vi "test_turbo1.vi"() -> ()   [LabVIEW 2018]
uses:
  <vilib>/addons/Modulation/Analog/support/mod_Set Error Source.vi
  <vilib>/addons/Modulation/Digital/Support/Common/Validators/mod_AWGN Validate.vi
  <vilib>/addons/Modulation/Digital/Impairments/subVIs/mod_createSeeds.vi
  <vilib>/addons/Modulation/Digital/Support/Common/Validators/mod_Validate Samples Per Symbol.vi
  <vilib>/addons/Modulation/Analog/support/Validators/mod_Validate Complex Waveform.vi
  <vilib>/addons/Modulation/Analog/support/Validators/mod_WFErrorHandler.vi
  <vilib>/addons/Modulation/Digital/Support/Common/Validators/mod_Generate Filter Coefficients Validate.vi
  <vilib>/addons/Modulation/Digital/General/subVIs/mod_Generate Filter Coefficients.vi
  <vilib>/addons/Modulation/Digital/General/MT Generate PSK System Parameters(M).vi
  <vilib>/addons/Modulation/Digital/General/subVIs/mod_Generate Bits PN Sequence.vi
  <vilib>/Analysis/1siggen.llb/Gaussian White Noise (obs 90).vi
  <vilib>/addons/Modulation/Digital/General/MT Apply Matched Filter (Generic).vi
  <vilib>/addons/Modulation/niDMT.lvlib
panel:
  out "size(s) 2":i32
  out "size(s)":i32
  out "%%%":i32
  out "****":i32
  out "ЁЁ":i32
  out "sortie turbocodeur":string
  out "BER":dbl
  in  "Eb/N0":dbl=10.0 format="%.2f"
  out "message":i8[](array[numeric])
  out "dec":i8[](array[numeric])
  out "sigma2":string
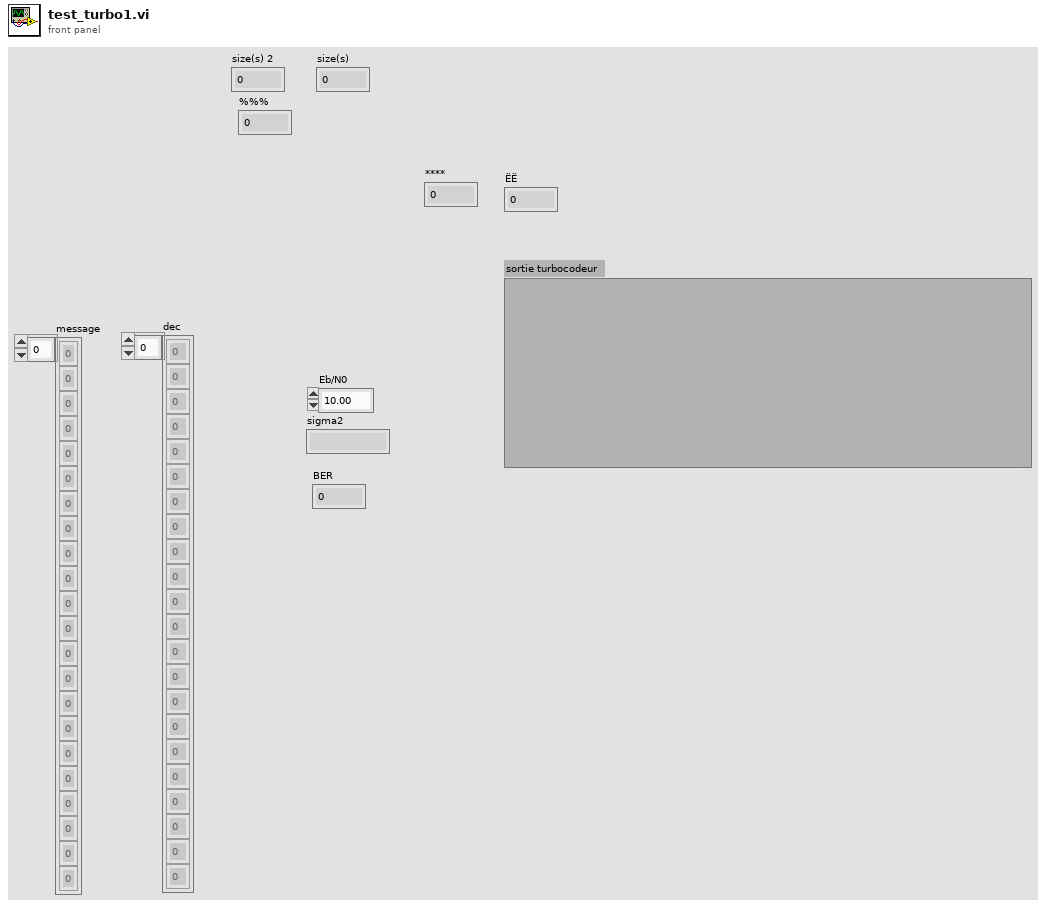
[diagram p1: front panel]
types:
  T1 = enum16{"none", "Raised Cosine", "Root Raised Cos", "Gaussian"}
  T2 = cluster{"samples per symbol (16)":i32, "symbol map":cdb[], "differential PSK":enum16{"disable", "enable"}, "PSK type":u16}
  T3 = typedef "niAMT.lvlib/Complex Data Waveform.ctl" = cluster{"t0":dbl, "dt":dbl, "Y":cdb[]}
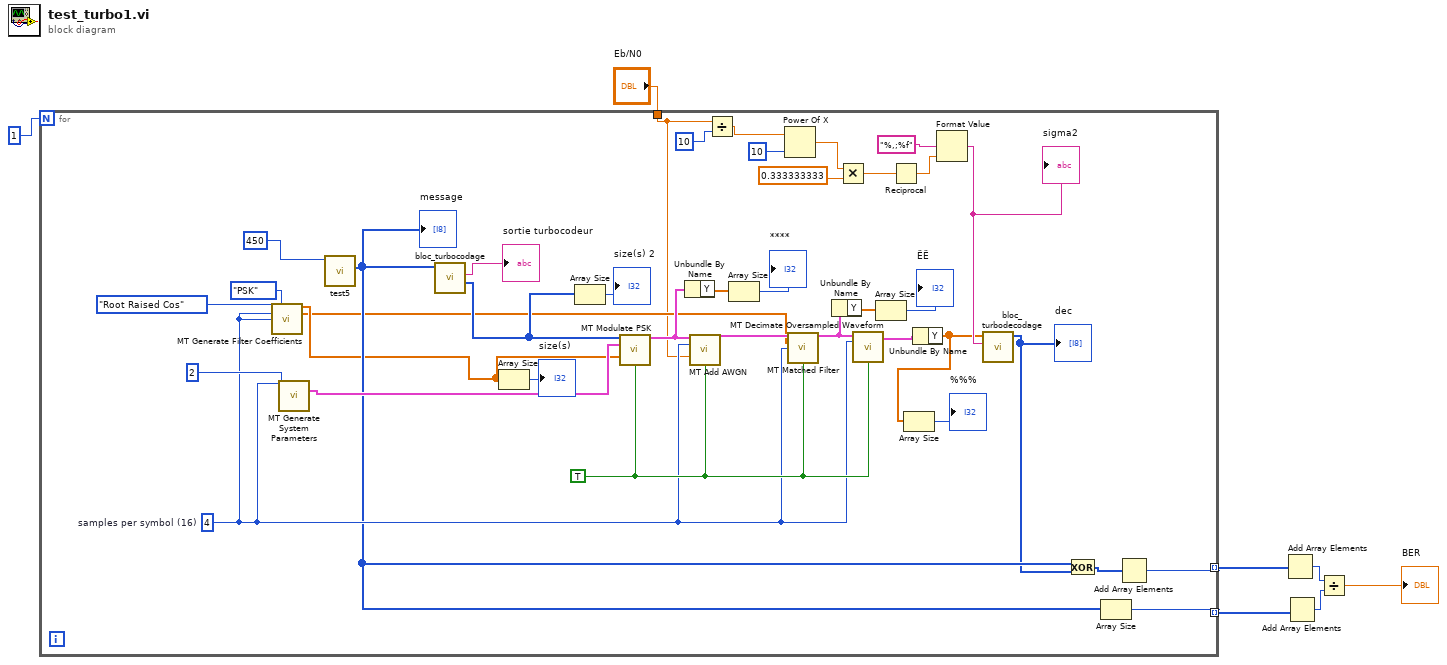
[diagram p0: block diagram]
diagram:
  n1 = for {
    N: 1 -> [_]
    tunnel: [w31] -> w5 mode=indexing
    tunnel: [w30] -> w4 mode=indexing
    tunnel: "Eb/N0" -> [w10]
    w38 = 4  # samples per symbol (16)
    w42 = TRUE ("reset? (T)")
    n2 = call <vilib>:"MT Generate Filter Coefficients.vi"("pulse shaping filter (none)"=T1."Root Raised Cos", "modulation type"=enum16{"FSK", "PSK", "QAM", "MSK", "PAM", "ASK"}."PSK", "pulse shaping samples per symbol (16)"=w38, "matched samples per symbol (16)"=w38) -> ("pulse shaping filter coefficients"=w16:dbl[], "matched filter coefficients"=w13:dbl[])  [unwired: 9 in, 1 out]
    n3 = call-poly <vilib>:"MT Generate System Parameters.vi"("samples per symbol (16)"=w38, "M-PSK (4)"=2) -> ("PSK system parameters"=w37:T2)  [unwired: 11 in, 2 out]
    n4 = call "test5.vi"("k"=450) -> ("output bit stream"=w29:i8[])  [unwired: 9 in, 1 out]
    "message" <- w29
    n5 = call "bloc_turbocodage.vi"("Array in"=w29) -> ("output bit stream"=w18:i8[], "sortie turbocodeur"=→"sortie turbocodeur":string)  [unwired: 8 in, 1 out]
    n6 = Array Size(array=w16) -> (size(s)=→"size(s)":i32)
    n7 = Array Size(array=w18) -> (size(s)=→"size(s) 2":i32)
    n8 = call <vilib>:"MT Modulate PSK.vi"("input bit stream"=w18, "PSK system parameters"=w37, "pulse shaping filter coefficients"=w16, "reset? (T)"=w42) -> ("output complex waveform"=w15:T3)  [unwired: 9 in, 2 out]
    n9 = Unbundle By Name(w15) -> ("Y"=w14:cdb[])
    n10 = call <vilib>:"MT Add AWGN.vi"("input complex waveform"=w15, "samples per symbol (16)"=w38, "Eb/N0 (10 dB)"=w10, "reset? (T)"=w42) -> ("output complex waveform"=w45:T3)  [unwired: 9 in, 2 out]
    n11 = Divide(x=w10, y=10) -> (x/y=w9:dbl)
    n12 = Array Size(array=w14) -> (size(s)=→"****":i32)
    n13 = Power Of X(1:10, 2:w9) -> (0:w11:dbl)
    n14 = call-poly <vilib>:"MT Matched Filter.vi"("input complex waveform"=w45, "matched filter coefficients"=w13, "samples per symbol (16)"=w38, "reset? (T)"=w42) -> ("output complex waveform"=w25:T3)  [unwired: 10 in, 1 out]
    n15 = Unbundle By Name(w25) -> ("Y"=w24:cdb[])
    n16 = Multiply(x=w11, y=0.333333333) -> (x*y=w35:dbl)
    n17 = call <vilib>:"MT Decimate Oversampled Waveform.vi"("input complex waveform"=w25, "decimation factor"=w38, "reset? (T)"=w42) -> ("output complex waveform"=w44:T3)  [unwired: 11 in, 1 out]
    n18 = Array Size(array=w24) -> (size(s)=→"ЁЁ":i32)
    n19 = Reciprocal(x=w35) -> (1/x=w33:dbl)
    n20 = Unbundle By Name(w44) -> ("Y"=w20:cdb[])
    n21 = Array Size(array=w20) -> (size(s)=→"%%%":i32)
    n22 = Format Value(format string="%,;%f", value (0)=w33) -> (output string=w27:string)  [unwired: 1 in]
    "sigma2" <- w27
    n23 = call "bloc_turbodecodage.vi"("sigma2"=w27, "Array"=w20) -> ("output bit stream"=w26:i8[])  [unwired: 7 in, 2 out]
    "dec" <- w26
    n24 = Exclusive Or(1:w26, 2:w29) -> (0:w32:i8[])
    n25 = Array Size(array=w29) -> (size(s)=w30:i32)
    n26 = Add Array Elements(numeric array=w32) -> (sum=w31:i8)
  }
  n27 = Add Array Elements(numeric array=w5) -> (sum=w3:i8)
  n28 = Add Array Elements(numeric array=w4) -> (sum=w2:i32)
  n29 = Divide(x=w3, y=w2) -> (x/y=→"BER":dbl)
